vi "GetFroshYear.vi"(8 "Error In":errorcluster) -> (0 "Error Out":errorcluster, 1 "Fall Term?":bool, 2 "Graduation Year":i8, 3 "Today's Date":string)   [LabVIEW 2015]
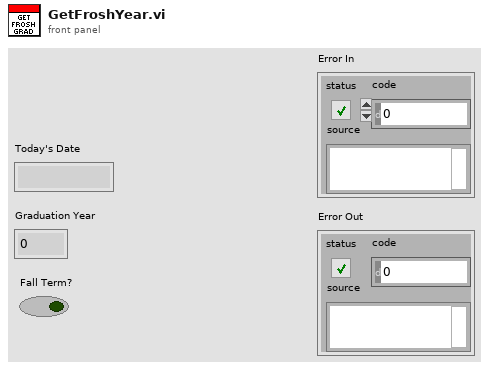
[diagram p1: front panel]
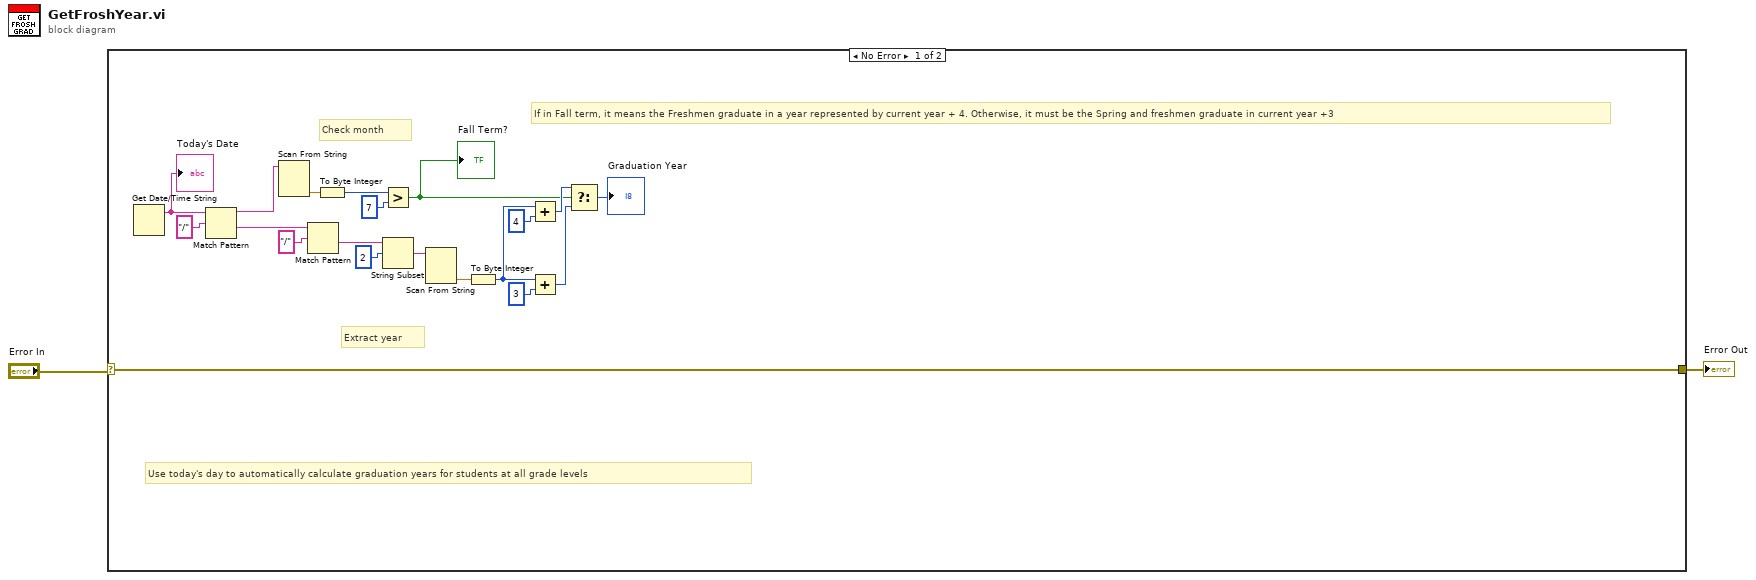
[diagram p0: block diagram]
diagram:
  n1 = case shown="No Error" "Error In" {
    selector: "Error In" -> [w3 w23]
    tunnel: [w3 w23] -> w1
    frame No Error {
      # "Extract year"
      # "Check month"
      # "Use today's day to automatically calculate graduation years for students at all grade levels"
      # "If in Fall term, it means the Freshmen graduate in a year represented by current year + 4. Otherwise, it must be the Spring and freshmen graduate in current year +3"
      n2 = Get Date/Time String() -> (date string=w22:string)  [unwired: 3 in, 1 out]
      "Today's Date" <- w22
      n3 = Match Pattern(string=w22, regular expression="/") -> (before substring=w5:string, after substring=w10:string)  [unwired: 1 in, 2 out]
      n4 = Scan From String(input string=w5) -> (output 1=w6:dbl)  [unwired: 4 in, 3 out]
      n5 = Match Pattern(string=w10, regular expression="/") -> (after substring=w11:string)  [unwired: 1 in, 3 out]
      n6 = To Byte Integer(number=w6) -> (8bit integer=w7:i8)
      n7 = Greater?(x=w7, y=i8 7) -> (0:w15:bool)
      "Fall Term?" <- w15
      n8 = String Subset(string=w11, offset (0)=2) -> (substring=w13:string)  [unwired: 1 in]
      n9 = Scan From String(input string=w13) -> (output 1=w14:dbl)  [unwired: 4 in, 3 out]
      n10 = To Byte Integer(number=w14) -> (8bit integer=w18:i8)
      n11 = Add(x=w18, y=i8 4) -> (x+y=w16:i8)
      n12 = Add(x=w18, y=i8 3) -> (x+y=w20:i8)
      n13 = Select(t=w16, s=w15, f=w20) -> (s? t:f=→"Graduation Year":i8)
    }
    frame Error {
    }
  }
  "Error Out" <- w1
